vi "testVerifyDerivedKey.vi"(8 "error in (no error)":errorcluster, 11 "TestCase in":refnum<class "TestPBKDF2.lvclass">) -> (0 "error out":errorcluster, 3 "TestCase out":refnum<class "TestPBKDF2.lvclass">)   [LabVIEW 2021, in "TestPBKDF2.lvclass"]
uses:
  TestPBKDF2.lvclass
  Source Code/Asymmetric Encryption/RSA/HashingAlgorithm.ctl
  <vilib>/addons/_JKI Toolkits/VI Tester/TestCase.llb/TestCase.lvclass
  Source Code/Key Derivation/dotNET Crypto Key Derivation.lvlib
  Source Code/Utility/dotNET Crypto Utility.lvlib
  C:/Program Files (x86)/National Instruments/LabVIEW 2021/vi.lib/addons/_JKI Toolkits/VI Tester/TestCase.llb/TestCase.lvclass
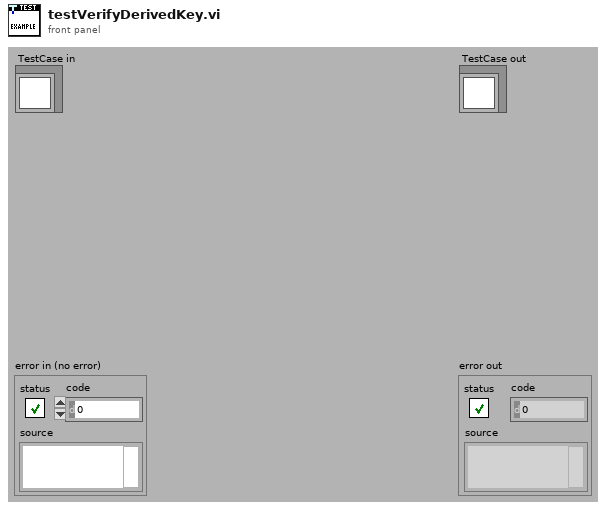
[diagram p1: front panel]
types:
  T1 = typedef "dotNET Crypto Utility.lvlib/HashingAlgorithm.ctl" = enum16{"MD5", "SHA1", "SHA256", "SHA384", "SHA512"}
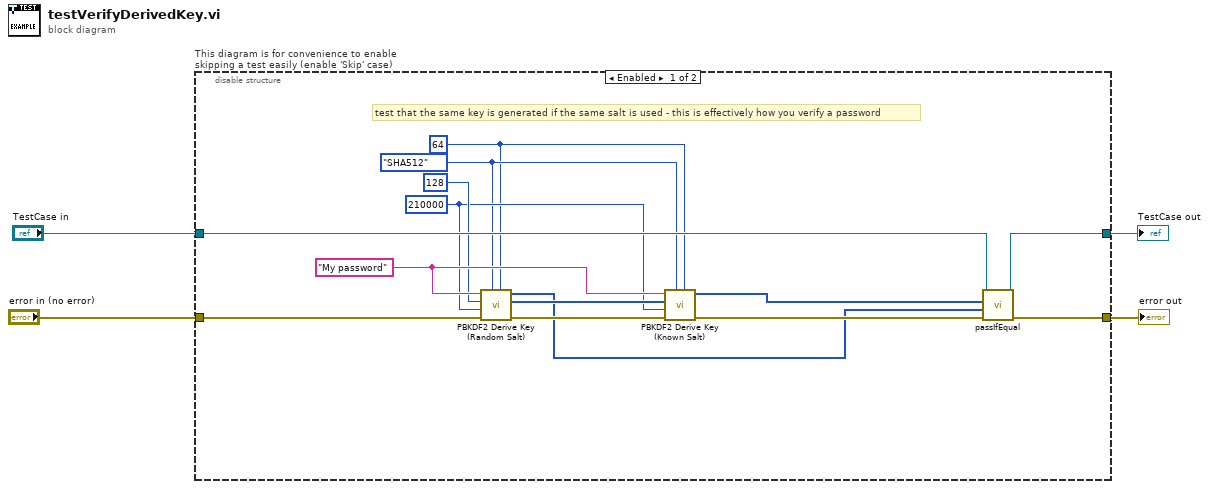
[diagram p0: block diagram]
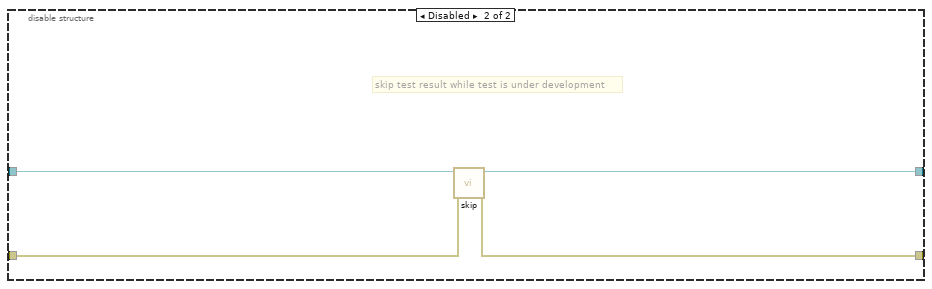
[diagram p2: hidden frame]
diagram:
  n1 = disable-structure "This diagram is for convenience to enable skipping a test easily (enable 'Skip' case)" shown="Enabled" {
    disable-tunnel: "TestCase in" -> [w18 w22]
    disable-tunnel: [w17 w20] -> w1
    disable-tunnel: [w16 w21] -> w3
    disable-tunnel: "error in (no error)" -> [w15 w19]
    frame Enabled {
      w12 = "My password" ("Password")
      w9 = 210000 ("iterations (210000)")
      w8 = HashingAlgorithm."SHA512" ("HashingAlgorithm (SHA512)")
      w7 = 64 ("Key length (64 bytes)")
      # "test that the same key is generated if the same salt is used - this is effectively how you verify a password"
      n2 = call "PBKDF2 Derive Key (Random Salt).vi"("Key length (64 bytes)"=w7, "HashingAlgorithm (SHA512)"=w8, "error in (no error)"=w15, "iterations (210000)"=w9, "saltSize (16 bytes)"=128 ("saltSize (128)"), "Password"=w12) -> ("error out"=w14:errorcluster, "Salt"=w10:u8[], "Derived Key"=w6:u8[])  [unwired: 3 in]
      n3 = call "PBKDF2 Derive Key (Known Salt).vi"("Key length (64 bytes)"=w7, "HashingAlgorithm (SHA512)"=w8, "error in (no error)"=w14, "iterations (210000)"=w9, "Salt"=w10, "Password"=w12) -> ("error out"=w13:errorcluster, "Derived Key"=w5:u8[])  [unwired: 4 in]
      n4 = call-dynamic "passIfEqual.vi"("error in (no error)"=w13, "y"=w6, "x"=w5, "TestCase in"=w18) -> ("error out"=w16:errorcluster, "TestCase out"=w17:refnum<class "TestPBKDF2.lvclass">)  [unwired: 6 in]
    }
    frame Disabled {
      # "skip test result while test is under development"
      n5 = call <vilib>:"skip.vi"("error in (no error)"=w19, "TestCase in"=w22) -> ("error out"=w21:errorcluster, "TestCase out"=w20:refnum<class "TestPBKDF2.lvclass">)  [unwired: 8 in]
    }
  }
  "error out" <- w3
  "TestCase out" <- w1
